vi "Zedver_v3_PrepCluster_DEFI.vi"(4 "PROCE CSV":path, 6 "HISTO CSV":path, 7 "Petición":T1="1", 8 "RAW CSV":path, 9 "Procesado":bool, 10 "Histograma":bool, 11 "RAW":bool) -> (1 "input cluster":T2, 3 "data string":string)   [LabVIEW 2011]
uses:
  Control 2.ctl
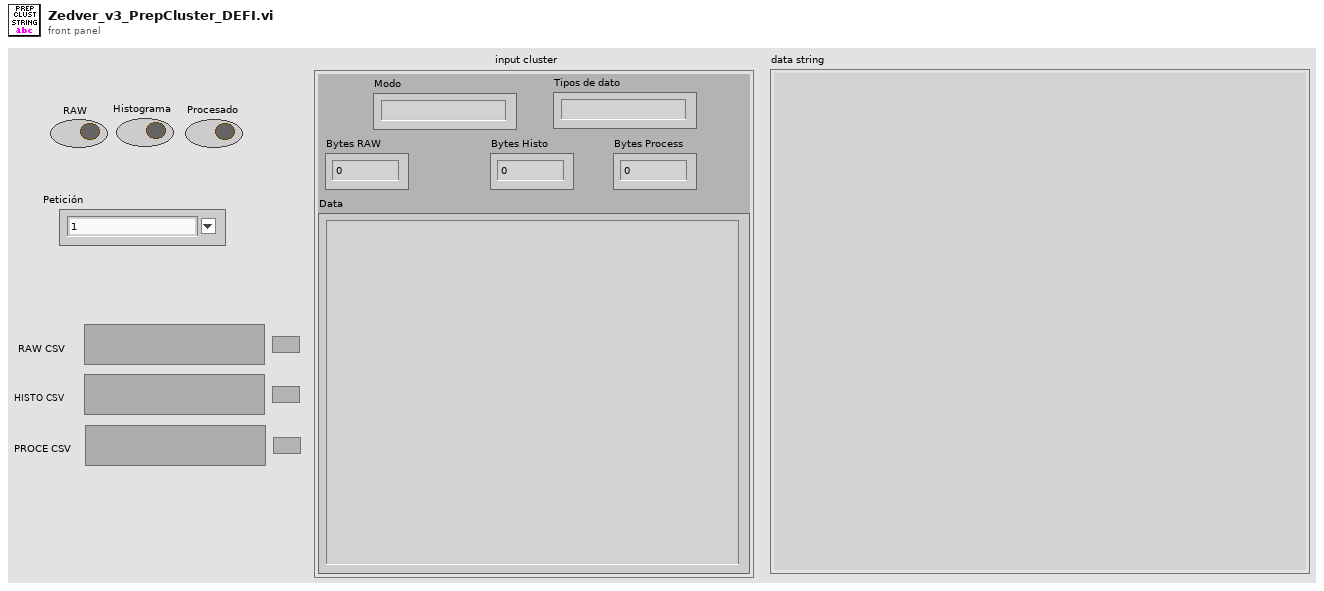
[diagram p1: front panel]
types:
  T1 = typedef "Control 2.ctl" = string
  T2 = cluster{"Modo":string, "Tipos de dato":string, "Bytes RAW":u16, "Bytes Histo":u16, "Bytes Process":u16, "Data":string}
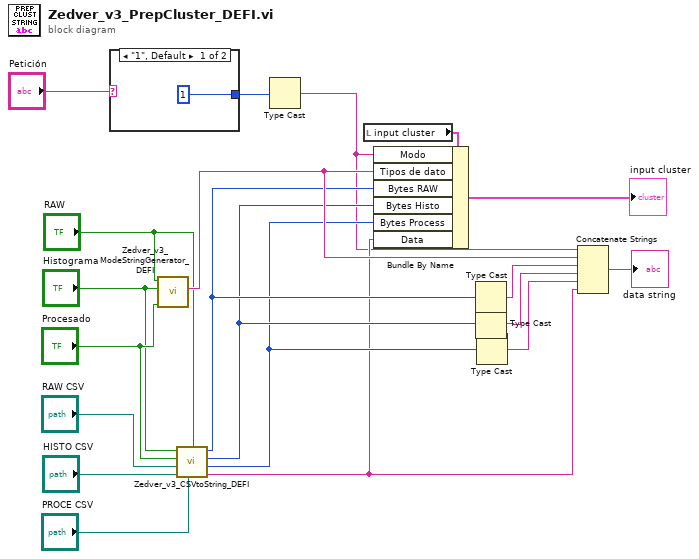
[diagram p0: block diagram]
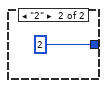
[diagram p2: hidden frame]
diagram:
  n1 = case shown="\"1\", Default" "Petición" {
    tunnel: [u8 1 u8 2] -> w2
    frame "1", Default {
    }
    frame "2" {
    }
  }
  n2 = call "Zedver_v3_ModeStringGenerator_DEFI.vi"("Procesado"="Procesado", "Histograma"="Histograma", "RAW"="RAW") -> ("decimal integer string"=w18:string)  [unwired: 8 in]
  n3 = call "Zedver_v3_CSVtoString_DEFI.vi"("PROCE CSV"="PROCE CSV", "RAW Activ."="RAW", "HISTO CSV"="HISTO CSV", "RAW CSV"="RAW CSV", "Process Activ."="Procesado", "Histogram Activ."="Histograma") -> ("concatenated string"=w3:string, "Process bytes"=w4:u16, "Histogram bytes"=w5:u16, "Raw bytes"=w6:u16)  [unwired: 2 in]
  n4 = Type Cast(x=w2) -> (*(type *) &x=w1:string)  [unwired: 1 in]
  n5 = local read "input cluster"() -> (w20:T2)
  n6 = Bundle By Name(cluster=w20, "Modo"=w1, "Tipos de dato"=w18, "Bytes RAW"=w6, "Bytes Histo"=w5, "Bytes Process"=w4, "Data"=w3) -> (→"input cluster":T2)
  n7 = Type Cast(x=w6) -> (*(type *) &x=w17:string)  [unwired: 1 in]
  n8 = Type Cast(x=w5) -> (*(type *) &x=w16:string)  [unwired: 1 in]
  n9 = Type Cast(x=w4) -> (*(type *) &x=w15:string)  [unwired: 1 in]
  n10 = Concatenate Strings(w1, w18, w17, w16, w15, w3) -> (→"data string":string)
